vi "화상키보드.vi"() -> ()   [LabVIEW 2014]
panel:
  in  "문자열":string
  in  "숫자형":dbl
  in  "화상 키보드":bool
  in  "정지":bool
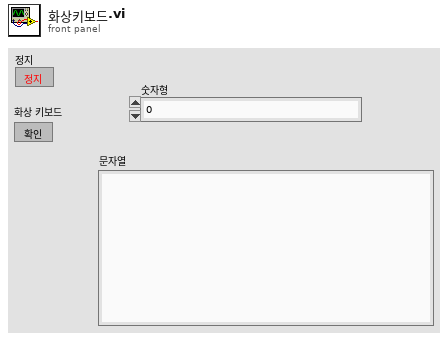
[diagram p1: front panel]
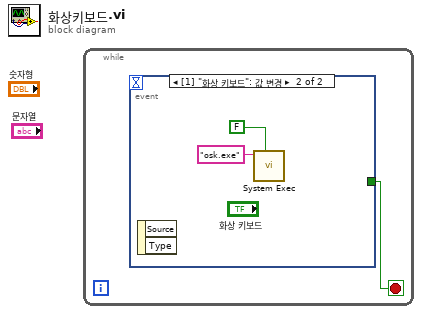
[diagram p0: block diagram]
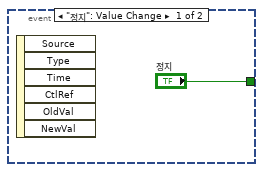
[diagram p2: hidden frame]
diagram:
  n1 = while {
    stop <- w1 stop-if-true
    n2 = event shown="[1] \"화상 키보드\": 값 변경" {
      selector: _ -> [_ _]
      dyn-events: _ -> [_ _]
      timeout: _ -> [_ _]
      tunnel: ["정지" _] -> w1
      event "정지": Value Change {
        n3 = event-data() -> ()  [unwired: 1 in, 6 out]
      }
      event "화상 키보드": Value Change {
        n4 = event-data() -> ()  [unwired: 1 in, 2 out]
        n5 = call <vilib>:"System Exec.vi"("wait until completion? (T)"=FALSE, "command line"="osk.exe") -> ()  [unwired: 6 in, 4 out]
      }
    }
  }
